vi "Begin.vi"(8 "error in":errorcluster) -> (0 "error out":errorcluster)   [LabVIEW 2017]
doc: "Called before other user functions, this VI is expected to open initial I/O refnums, load in file data, and do all program initialization. Notice that the <B>error out</B> terminal is simply used for data flow. Wiring it to other structures or subVIs ensures that this VI runs first."
uses:
  <vilib>/Rock Robotics/WPI/DriverStation/WPI_DriverStationRobotMode2.ctl
  Robot Global Data.vi
  <vilib>/Rock Robotics/Network Tables/NT Write String Array.vi
  981LabViewComponents/Telop Counter Variable.vi
  981LabViewComponents/Joystick 2 Trigger.vi
  981LabViewComponents/Global Simulated Arm Pot.vi
  <vilib>/Rock Robotics/WPI/ThirdParty/Sensors/navX/_Processing Loop/FRIC_navX_Internal_I2C_ProcessingLoop.vi
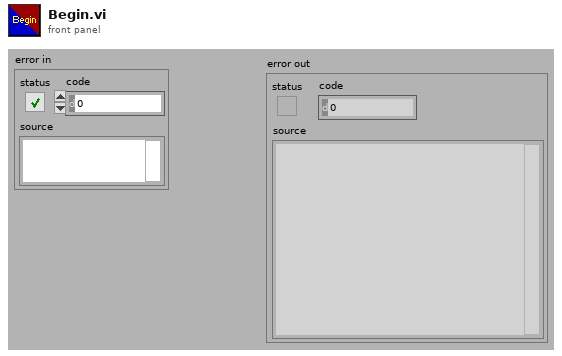
[diagram p1: front panel]
types:
  T1 = typedef "WPI_DriverStationRobotMode2.ctl" = enum16{"Autonomous Disabled", "Autonomous Enabled", "Teleop Disabled", "Teleop Enabled", "Disconnected", "Finish", "Test Disabled", "Test Enabled", "Emergency Stopped"}
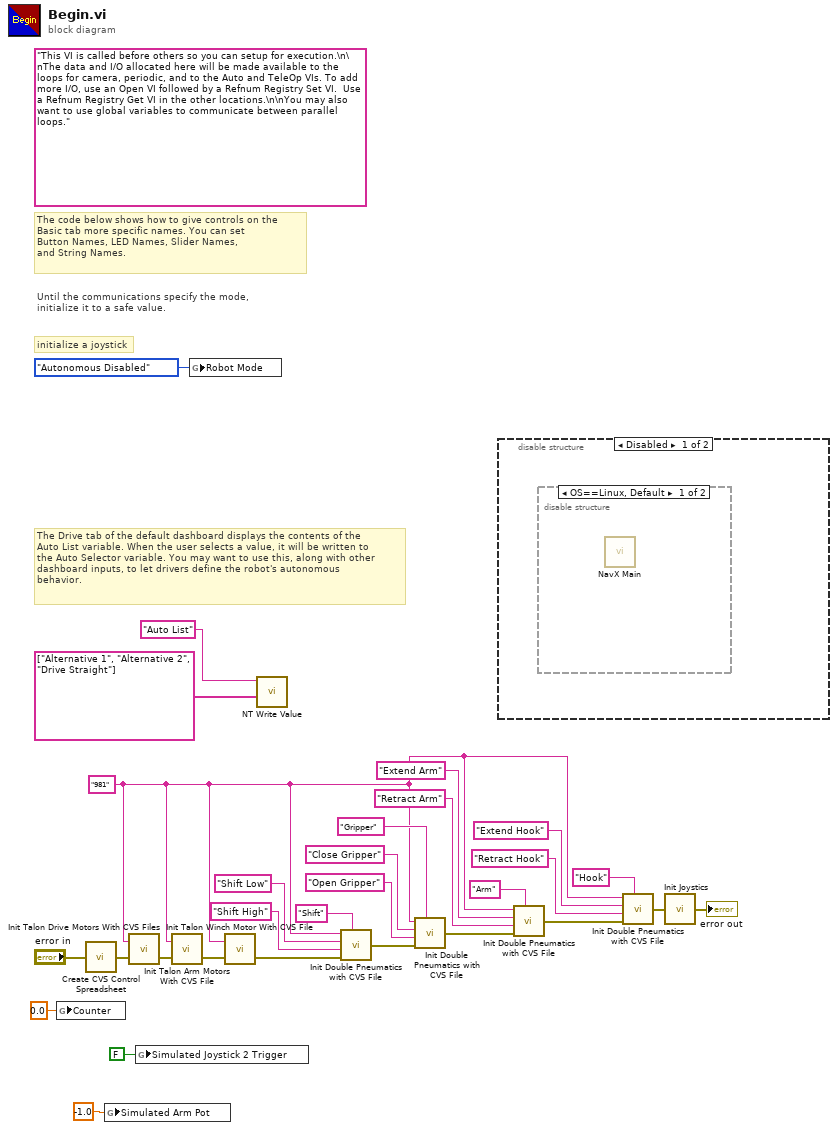
[diagram p0: block diagram]
diagram:
  w9 = "981" ("Robot ID")
  (unwired) "This VI is called before others so you can setup for execution.\n\nThe data and I/O allocated here will be made available to the loops for camera, periodic, and to the Auto and TeleOp VIs. To add more I/O, use an Open VI followed by a Refnum Registry Set VI.  Use a Refnum Registry Get VI in the other locations.\n\nYou may also want to use global variables to communicate between parallel loops."
  # "The Drive tab of the default dashboard displays the contents of the\nAuto List variable. When the user selects a value, it will be written to\nthe Auto Selector variable. You may want to use this, along with other\ndashboard inputs, to let drivers define the robot's autonomous\nbehavior."
  # "The code below shows how to give controls on the\nBasic tab more specific names. You can set\nButton Names, LED Names, Slider Names,\nand String Names."
  # "initialize a joystick"
  # "Until the communications specify the mode,\ninitialize it to a safe value."
  n1 = global write "Telop Counter Variable.vi" "Counter"(0.0 ("Counter")) -> ()
  n2 = call "Create CVS Control Spreadsheet.vi"("error in"="error in") -> ("error out"=w16:errorcluster)
  n3 = global write "Global Simulated Arm Pot.vi" "Simulated Arm Pot"(-1.0 ("Simulated Arm Pot")) -> ()
  n4 = call "Init Talon Drive Motors With CVS Files.vi"("error in"=w16, "Robot ID"=w9) -> ("error out"=w15:errorcluster)  [unwired: 1 out]
  n5 = global write "Joystick 2 Trigger.vi" "Simulated Joystick 2 Trigger"(FALSE ("Trigger")) -> ()
  n6 = call "Init Talon Arm Motors With CVS File.vi"("error in"=w15, "Robot ID"=w9) -> ("error out"=w14:errorcluster)  [unwired: 1 out]
  n7 = global write "Robot Global Data.vi" "Robot Mode"(WPI_DriverStationRobotMode2."Autonomous Disabled" ("Robot Mode")) -> ()
  n8 = call "Init Talon Winch Motor With CVS File.vi"("error in"=w14, "Robot ID"=w9) -> ("error out"=w12:errorcluster)  [unwired: 1 out]
  n9 = call-poly <vilib>:"NT Write Value.vi"("String Array"=string[] ["Alternative 1", "Alternative 2", "Drive Straight"], "Name"="Auto List") -> ()  [unwired: 9 in, 1 out]
  n10 = call "Init Double Pneumatics with CVS File.vi"("Robot ID"=w9, "Forward Pnumatic ID"="Shift Low" ("Motor ID"), "Reverse Pnumatic ID"="Shift High", "error in"=w12, "Actuator Name"="Shift") -> ("error out"=w11:errorcluster)
  n11 = call "Init Double Pneumatics with CVS File.vi"("Robot ID"=w9, "Forward Pnumatic ID"="Close Gripper" ("Motor ID"), "Reverse Pnumatic ID"="Open Gripper", "error in"=w11, "Actuator Name"="Gripper") -> ("error out"=w10:errorcluster)
  n12 = disable-structure shown="Disabled" {
    frame Disabled {
      n13 = disable-structure shown="OS==Linux, Default" {
        frame condition #0 (active) {
          n14 = call-poly <vilib>:"NavX Main.vi"() -> ()  [unwired: 12 in]
        }
        frame condition #1 {
        }
      }
    }
    frame Enabled {
    }
  }
  n15 = call "Init Double Pneumatics with CVS File.vi"("Robot ID"=w9, "Forward Pnumatic ID"="Extend Arm" ("Motor ID"), "Reverse Pnumatic ID"="Retract Arm", "error in"=w10, "Actuator Name"="Arm") -> ("error out"=w5:errorcluster)
  n16 = call "Init Double Pneumatics with CVS File.vi"("Robot ID"=w9, "Forward Pnumatic ID"="Extend Hook", "Reverse Pnumatic ID"="Retract Hook", "error in"=w5, "Actuator Name"="Hook") -> ("error out"=w4:errorcluster)
  n17 = call "Init Joystics.vi"("error in"=w4) -> ("error out"=→"error out":errorcluster)
